vi "624WPI_CameraGet Image From TCP.vi"(7 "Camera Mode":u16(ring) items=["Camera Off", "USB Camera SW", "USB Camera HW", "IP Camera"], 8 "error in (no error)":errorcluster, 9 "USB":bool, 10 "Image In":T1, 11 "connection ID":refnum<k5>) -> (0 "error out":errorcluster, 1 "Size":i32, 2 "Image Out":T1, 3 "connection ID (dup)":refnum<k5>)   [LabVIEW 2014]
doc: "This software is licensed. Open the labview\\readme\\WPI Robotics Library Open Source License.txt file for more information."
uses:
  <vilib>/vision/Image Controls.llb/IMAQ Image.ctl
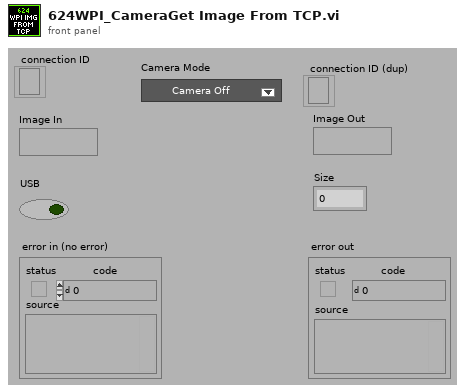
[diagram p1: front panel]
types:
  T1 = typedef "IMAQ Image.ctl" = refnum<image>
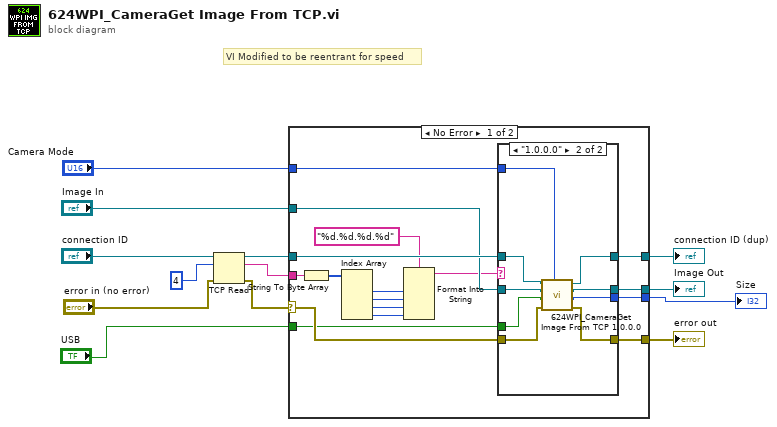
[diagram p0: block diagram]
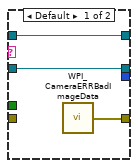
[diagram p2: hidden frame]
diagram:
  # "VI Modified to be reentrant for speed"
  n1 = TCP Read(connection ID="connection ID", bytes to read=4, error in (no error)="error in (no error)") -> (connection ID out=w13:refnum<k5>, data out=w9:string, error out=w4:errorcluster)  [unwired: 2 out]
  n2 = case shown="No Error" w4 {
    selector: w4 -> [w17 w43]
    tunnel: w13 -> [w30 w45]
    tunnel: "Image In" -> [w29 w44]
    tunnel: w9 -> [w22 _]
    tunnel: [w20 w43] -> w7
    tunnel: [w19 w44] -> w6
    tunnel: [w18 w45] -> w5
    tunnel: "USB" -> [w16 _]
    tunnel: [w15 _] -> w2
    tunnel: "Camera Mode" -> [w14 _]
    frame No Error {
      n3 = String To Byte Array(string=w22) -> (unsigned byte array=w23:u8[])
      n4 = Index Array(array=w23) -> (element #1=w25:u8, element #2=w26:u8, element #3=w27:u8, element #4=w28:u8)  [unwired: 4 in]
      n5 = Format Into String(format string="%d.%d.%d.%d", w25, w26, w27, w28) -> (resulting string=w21:string)  [unwired: 2 in, 1 out]
      n6 = case shown="\"1.0.0.0\"" w21 {
        tunnel: w30 -> [w33 w35]
        tunnel: w29 -> [w32 w36]
        tunnel: w17 -> [_ w38]
        tunnel: [w31 w39] -> w20
        tunnel: [w32 w41] -> w19
        tunnel: [w33 w42] -> w18
        tunnel: w16 -> [_ w37]
        tunnel: [_ w40] -> w15
        tunnel: w14 -> [_ w34]
        frame Default {
          n7 = call <vilib>:"WPI_CameraERRBadImageData.vi"() -> ("error out"=w31:errorcluster)
        }
        frame "1.0.0.0" {
          n8 = call "624WPI_CameraGet Image From TCP 1.0.0.0.vi"("Camera Mode"=w34, "error in (no error)"=w38, "USB"=w37, "Image In"=w36, "connection ID"=w35) -> ("error out"=w39:errorcluster, "Size"=w40:i32, "Image Out"=w41:T1, "connection ID out"=w42:refnum<k5>)  [unwired: 3 in]
        }
      }
    }
    frame Error {
    }
  }
  "error out" <- w7
  "Image Out" <- w6
  "connection ID (dup)" <- w5
  "Size" <- w2
